vi "TimeScale.vi"() -> ()   [LabVIEW 2014]
uses:
  <vilib>/Analysis/NI_AALPro.lvlib
panel:
  in  "Function Inputs":cluster{"frequency":dbl, "# of samples":i32}={"frequency"=10.0, "# of samples"=100} {"frequency" scale=0.0..500.0}
  in  "Select Input type":string(combo)
  in  "signal type":T1(ring)
  out "graph of X(w/a)":cluster{"-pi to pi":dbl[], dbl[]}(graph)
  out "graph of DTFT{x(an)}":cluster{"-pi to pi":dbl[], "DTFT op":dbl[]}(graph)
  out "graph of x(n)":dbl[](graph)
  out "graph of x(an)":dbl[](graph)
  in  "Boolean":bool
  in  "Scaling factor":dbl
  out "x(an)":dbl[](array[numeric])
  in  "x(n)":dbl[](array[numeric])
  # "Instructions"
  # "If,\n        DTFT{x(n)} ----> X(w)\nthen, \n      DTFT{x(an)} ----> X(w/a)"
  # "1. Select the type of input\n2. In case of function generator, Select the signal type\n3. input the frequency and no. of samples\n4. input the scaling factor(>0)\n5. Check for the output and verify with theoretical value"
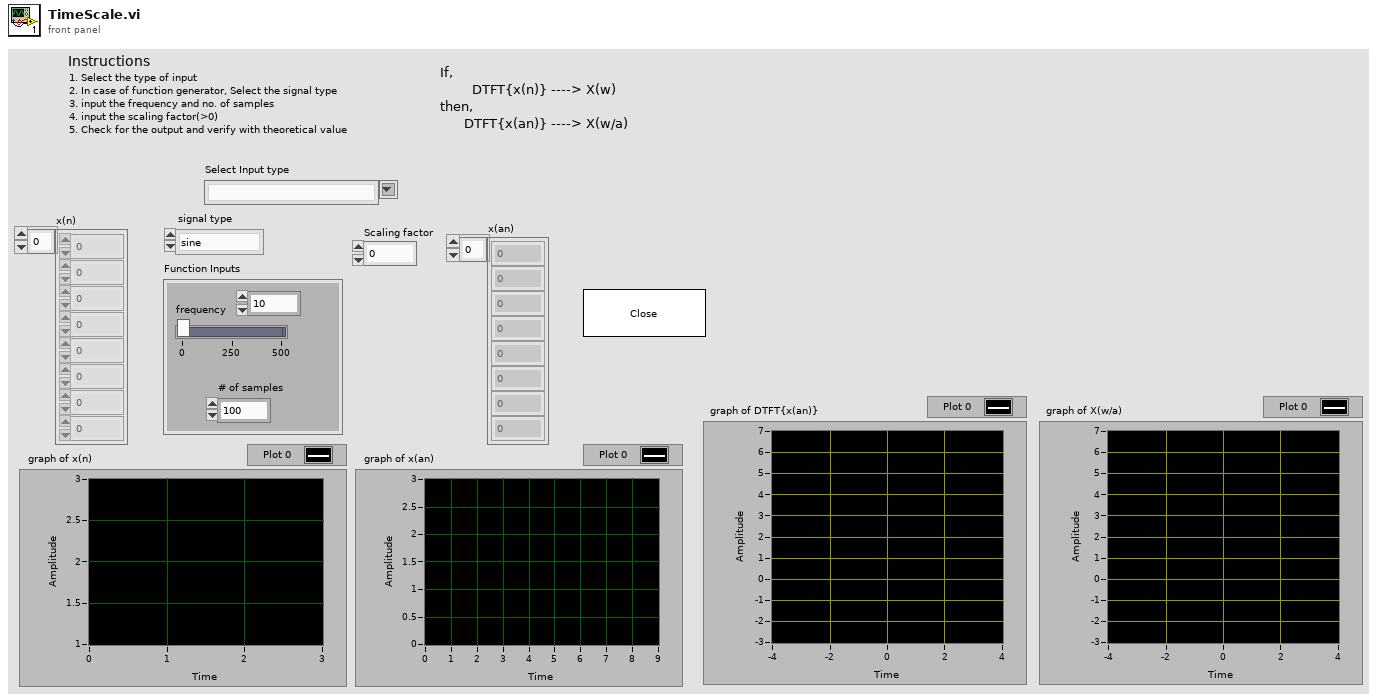
[diagram p1: front panel]
types:
  T1 = enum16{"sine", "cosine", "triangle", "square", "sawtooth", "increasing ramp", "decreasing ramp"}
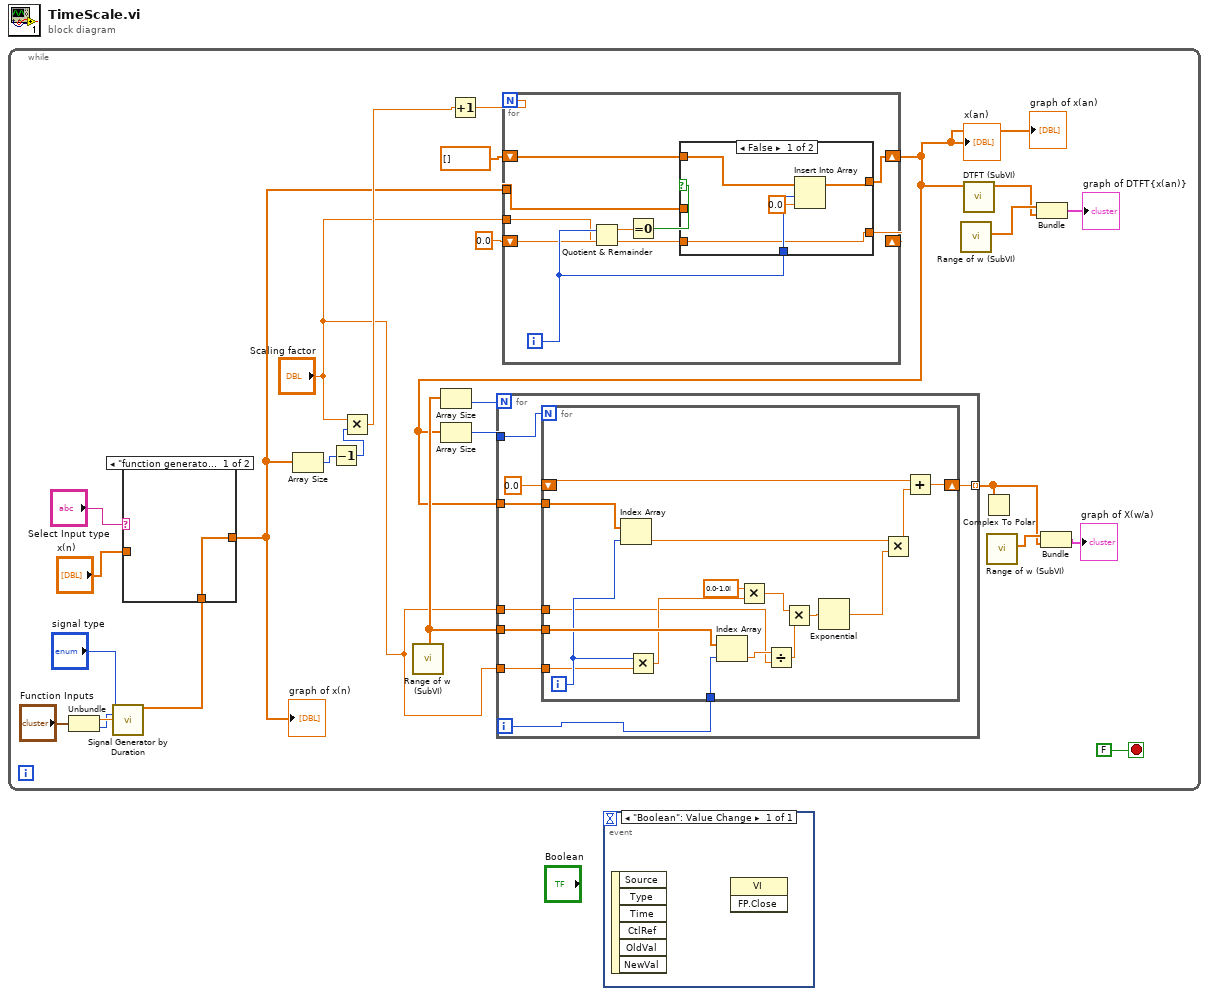
[diagram p0: block diagram]
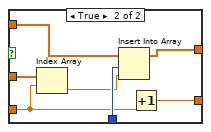
[diagram p3: hidden frame]
diagram:
  n1 = while {
    stop <- FALSE stop-if-true
    n2 = Unbundle("Function Inputs") -> ("frequency"=w2:dbl, "# of samples"=w1:i32)
    n3 = call <vilib>:"Signal Generator by Duration.vi"("signal type"="signal type", "# of samples"=w1, "frequency"=w2) -> ("signal"=w5:dbl[])  [unwired: 9 in, 3 out]
    n4 = case shown="\"function generator\", Default" "Select Input type" {
      tunnel: "x(n)" -> [_ w28]
      tunnel: w5 -> [w27 _]
      tunnel: [w27 w28] -> w4
      frame "function generator", Default {
      }
      frame "array" {
      }
    }
    "graph of x(n)" <- w4
    n5 = Array Size(array=w4) -> (size(s)=w17:i32)
    n6 = Decrement(x=w17) -> (x-1=w18:i32)
    n7 = Multiply(x="Scaling factor", y=w18) -> (x*y=w22:dbl)
    n8 = call "Range of w (SubVI).vi"() -> ("-pi to pi"=w23:dbl[])  [unwired: 11 in]
    n9 = Array Size(array=w23) -> (size(s)=w25:i32)
    n10 = Increment(x=w22) -> (x+1=w21:dbl)
    n11 = for {
      N: w21 -> [_]
      shift-right: [w36] -> w16
      shift-left: dbl[] [] -> [w35]
      tunnel: w4 -> [w30]
      shift-right: [w32] -> _
      shift-left: 0.0 -> [w31]
      tunnel: "Scaling factor" -> [w29]
      i -> [w33]
      n12 = Quotient & Remainder(x=w33, y=w29) -> (x-y*floor(x/y)=w34:dbl)  [unwired: 1 out]
      n13 = Equal To 0?(x=w34) -> (x = 0?=w37:bool)
      n14 = case shown="False" w37 {
        tunnel: [w40 w48] -> w36
        tunnel: w33 -> [w42 w49]
        tunnel: w35 -> [w39 w47]
        tunnel: [w38 w46] -> w32
        tunnel: w31 -> [w38 w45]
        tunnel: w30 -> [_ w44]
        frame False {
          n15 = Insert Into Array(array=w39, index=w42, new element=0.0 ("new element/subarray")) -> (w40:dbl[])
        }
        frame True {
          n16 = Index Array(array=w44, index=w45) -> (element=w43:dbl)
          n17 = Insert Into Array(array=w47, index=w49, new element=w43) -> (w48:dbl[])
          n18 = Increment(x=w45) -> (x+1=w46:dbl)
        }
      }
    }
    "x(an)" <- w16
    "graph of x(an)" <- w16
    n19 = Array Size(array=w16) -> (size(s)=w26:i32)
    n20 = for {
      N: w25 -> [_]
      tunnel: w23 -> [w57]
      tunnel: w26 -> [w56]
      tunnel: w16 -> [w54]
      tunnel: [w53] -> w13 mode=indexing
      tunnel: "Scaling factor" -> [w51]
      tunnel: "Scaling factor" -> [w50]
      i -> [w52]
      n21 = for {
        N: w56 -> [_]
        tunnel: w57 -> [w73]
        shift-right: [w68] -> w53
        shift-left: 0.0 -> [w67]
        tunnel: w54 -> [w65]
        tunnel: w52 -> [w64]
        tunnel: w51 -> [w59]
        tunnel: w50 -> [w58]
        i -> [w61]
        n22 = Index Array(array=w65, index=w61) -> (element=w66:dbl)
        n23 = Multiply(x=w61, y=w59) -> (x*y=w60:dbl)
        n24 = Index Array(array=w73, index=w64) -> (element=w63:dbl)
        n25 = Multiply(x=cdb 0.0-1.0i, y=w60) -> (x*y=w72:cdb)
        n26 = Divide(x=w63, y=w58) -> (x/y=w62:dbl)
        n27 = Multiply(x=w72, y=w62) -> (x*y=w71:cdb)
        n28 = Exponential(1:w71) -> (0:w70:cdb)
        n29 = Multiply(x=w66, y=w70) -> (x*y=w69:cdb)
        n30 = Add(x=w67, y=w69) -> (x+y=w68:cdb)
      }
    }
    n31 = call "Range of w (SubVI).vi"() -> ("-pi to pi"=w12:dbl[])  [unwired: 11 in]
    n32 = call "DTFT (SubVI).vi"("ip array"=w16) -> ("DTFT op"=w11:cdb[])  [unwired: 9 in, 1 out]
    n33 = Complex To Polar(r * e^(i*theta)=w13) -> ()  [unwired: 2 out]
    n34 = call "Range of w (SubVI).vi"() -> ("-pi to pi"=w14:dbl[])  [unwired: 11 in]
    n35 = Bundle("-pi to pi"=w12, "DTFT op"=w11) -> (→"graph of DTFT{x(an)}":cluster{"-pi to pi":dbl[], "DTFT op":cdb[]})  [unwired: 1 in]
    n36 = Bundle("-pi to pi"=w14, w13) -> (→"graph of X(w/a)":cluster{"-pi to pi":dbl[], cdb[]})  [unwired: 1 in]
  }
  n37 = event shown="[0] \"Boolean\": Value Change" {
    selector: _ -> [_]
    dyn-events: _ -> [_]
    timeout: _ -> [_]
    event "Boolean": Value Change {
      n38 = event-data() -> ()  [unwired: 1 in, 6 out]
      n39 = invoke class="VI" method="FP.Close"() -> ()  [unwired: 3 in, 3 out]
    }
  }
